vi "SSC DCPower Configure Voltage Level.vi"(0 "DCPower SSC in":T1[](array[typedef]), 5 "Voltage Level (V)":dbl format="%#_6p", 11 "error in":errorcluster) -> (4 "DCPower SSC out":T1[](array[typedef]), 15 "error out":errorcluster)   [LabVIEW 2020]
doc: "This VI configures the Voltage Level.\n\nThis can be used when in the single point voltage mode."
uses:
  SSC DCPower.ctl
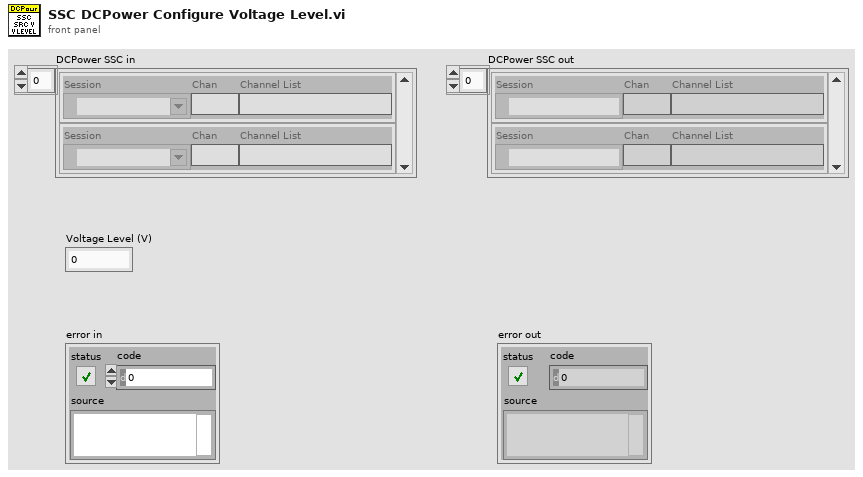
[diagram p1: front panel]
types:
  T1 = typedef "SSC DCPower.ctl" = cluster{"Session":refnum<k15>, "Chan":string, "Channel List":string}
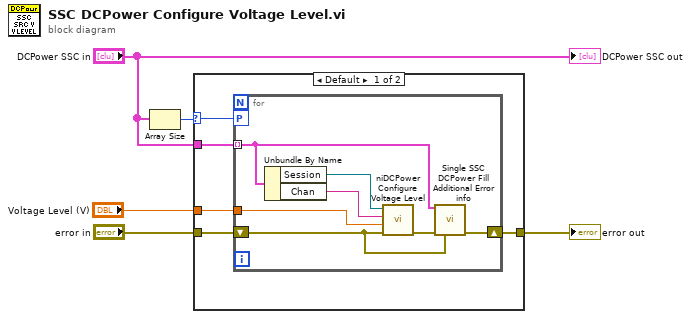
[diagram p0: block diagram]
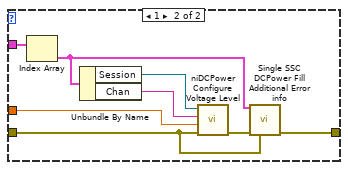
[diagram p2: hidden frame]
diagram:
  n1 = Array Size(array="DCPower SSC in") -> (size(s)=w2:i32)
  n2 = case shown="Default" w2 {
    selector: w2 -> [w7 _]
    tunnel: [w10 w25] -> w5
    tunnel: "error in" -> [w9 w24]
    tunnel: "Voltage Level (V)" -> [w8 w23]
    tunnel: "DCPower SSC in" -> [w6 w22]
    frame Default {
      n3 = for {
        tunnel: w6 -> [w12] mode=indexing
        workers-P: w7 -> [_]
        tunnel: w8 -> [w16]
        shift-right: [w13] -> w10
        shift-left: w9 -> [w11]
        n4 = Unbundle By Name(w12) -> ("Session"=w15:refnum<k15>, "Chan"=w14:string)
        n5 = call <instrlib>:"niDCPower Configure Voltage Level.vi"("error in (no error)"=w11, "voltage level"=w16, "channel name"=w14, "instrument handle"=w15) -> ("error out"=w17:errorcluster)  [unwired: 6 in, 1 out]
        n6 = call "Single SSC DCPower Fill Additional Error info.vi"("DCPower SSC in"=w12, "error in"=w17, "previous error in"=w11) -> ("error out"=w13:errorcluster)  [unwired: 12 in]
      }
    }
    frame 1 {
      n7 = Index Array(array=w22) -> (element=w18:T1)  [unwired: 1 in]
      n8 = Unbundle By Name(w18) -> ("Session"=w20:refnum<k15>, "Chan"=w19:string)
      n9 = call <instrlib>:"niDCPower Configure Voltage Level.vi"("error in (no error)"=w24, "voltage level"=w23, "channel name"=w19, "instrument handle"=w20) -> ("error out"=w21:errorcluster)  [unwired: 6 in, 1 out]
      n10 = call "Single SSC DCPower Fill Additional Error info.vi"("DCPower SSC in"=w18, "error in"=w21, "previous error in"=w24) -> ("error out"=w25:errorcluster)  [unwired: 12 in]
    }
  }
  "error out" <- w5
  "DCPower SSC out" <- "DCPower SSC in"
